vi "Pfeiffer-RVC300.get mode.vi"(0 "i ref in":refnum<vi>, 3 "ms timeout (10000)":i32=10000, 5 "error in (no error)":errorcluster) -> (14 "i ref out":refnum<vi>, 15 "regulationMode":T1, 17 "timed out":bool, 19 "error out":errorcluster)   [LabVIEW 2014, in "Pfeiffer-RVC300.lvlib"]
doc: "Gets the regulation mode from device (possible values: unknown / pressure / flow / wait).\n\nLicense Agreement for this software:\n\nCopyright (C)\nMax-Planck-Institut für Kernphysik\nSaupfercheckweg 1\n69117 Heidelberg\nGermany\n\nContact: christopher.borgmann@mpi-hd.mpg.de\n\nThis program is free software: you can redistribute it and/or modify \nit under the terms of the GNU General Public License as published by\nthe Free Software Foundation, either version 3 of the License, or\n(at your option) any later version.\n\nThis program is distributed in the hope that it will be useful,\nbut WITHOUT ANY WARRANTY; without even the implied warranty of\nMERCHANTABILITY or FITNESS FOR A PARTICULAR PURPOSE. See the\nGNU General Public License for more details.\n\nYou should have received a copy of the GNU General Public License\nalong with this program. If not, see <http://www.gnu.org/licenses/>.\n\nMax-Planck-Institut für Kernphysik\nSaupfercheckweg 1, 69117 Heidelberg, Germany\nFor all questions and ideas contact: christopher.borgmann@mpi-hd.mpg.de\nLast update: 08.07.2010"
uses:
  Pfeiffer-RVC300.lvlib
  CSCore/CSApplicationBaseClasses/DeviceBase/DeviceBase.lvlib
  Pfeiffer-RVC300.regulation mode.ctl
  CSlibraries-extern/DimLVEvent/LVDimInterface/LVDimInterface.lvlib
  CSlibraries/UtilityLib/UtilityLib.lvlib
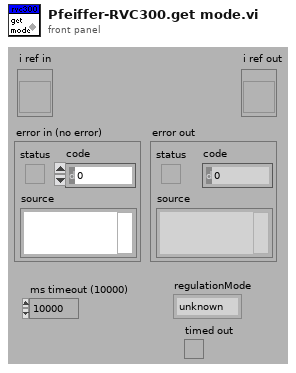
[diagram p1: front panel]
types:
  T1 = typedef "Pfeiffer-RVC300.lvlib/Pfeiffer-RVC300.regulation mode.ctl" = enum16{"unknown", "Pressure", "Flow", "Wait"}
  T2 = typedef "Pfeiffer-RVC300.lvlib/Pfeiffer-RVC300.i attribute.ctl" = cluster{"interfaceInitialized":bool, "VISAResource":refnum<visa-resource-name>, "WaitingTime":u32, "nomValues":T3, "actValues":T3}
  T3 = typedef "Pfeiffer-RVC300.lvlib/Pfeiffer-RVC300.parameters.ctl" = cluster{"regulationMode":T1, "valveType":string, "sensorType":string, "valveState":string, "flow":dbl, "pressure":dbl, "serviceIDs":cluster{"regulationModeID":i32, "valveTypeID":i32, "sensorTypeID":i32, "valveStateID":i32, "flowID":i32, "pressureID":i32}}
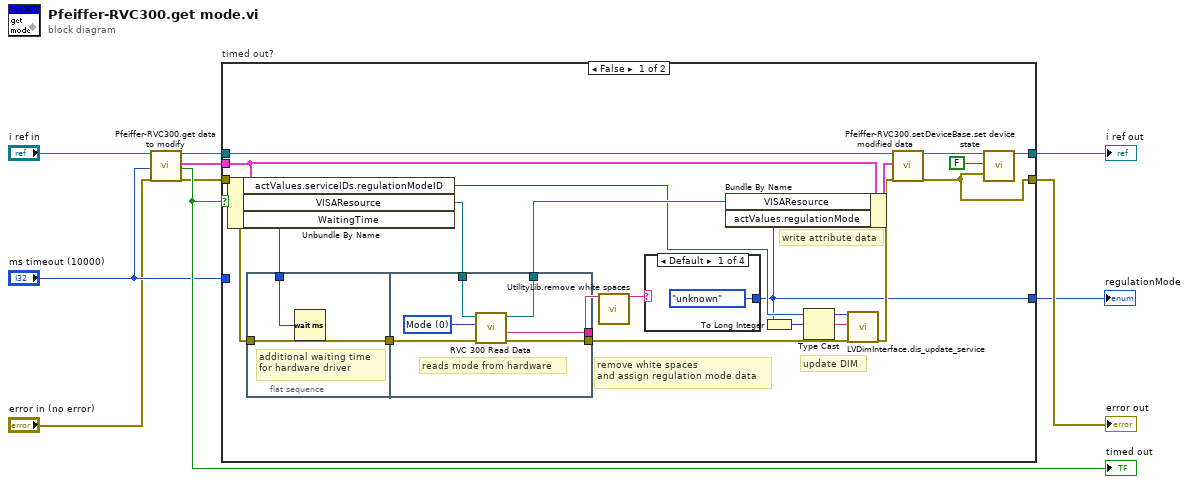
[diagram p0: block diagram]
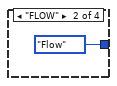
[diagram p2: hidden frame]
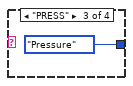
[diagram p3: hidden frame]
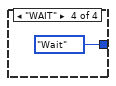
[diagram p4: hidden frame]
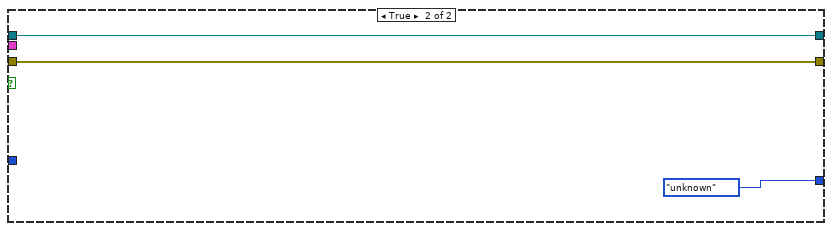
[diagram p5: hidden frame]
diagram:
  n1 = call "Pfeiffer-RVC300.get data to modify.vi"("i ref in"="i ref in", "ms timeout (10000)"="ms timeout (10000)", "error in (no error)"="error in (no error)") -> ("i ref out"=w4:refnum<vi>, "i attribute"=w2:T2, "timed out"=w7:bool, "error out"=w3:errorcluster)  [unwired: 13 in]
  "timed out" <- w7
  n2 = case "timed out?" shown="False" w7 {
    tunnel: [w27 w45] -> w9
    tunnel: w4 -> [w30 w45]
    tunnel: [w25 w44] -> w8
    tunnel: w3 -> [w24 w44]
    tunnel: w2 -> [w22 _]
    tunnel: "ms timeout (10000)" -> [_ _]
    tunnel: [w14 Pfeiffer-RVC300.regulation_mode."unknown" ("regulationMode 2")] -> w1
    frame False {
      # "write attribute data"
      # "remove white spaces\nand assign regulation mode data"
      # "update DIM"
      n3 = Unbundle By Name(w22) -> ("actValues.serviceIDs.regulationModeID"=w17:i32, "VISAResource"=w19:refnum<visa-resource-name>, "WaitingTime"=w20:u32)
      n4 = flat-sequence {
        tunnel: w24 -> [w36]
        tunnel: [w36] -> w23
        tunnel: w20 -> [w35]
        tunnel: w23 -> [w40]
        tunnel: w19 -> [w42]
        tunnel: [w39] -> w16
        tunnel: [w41] -> w21
        tunnel: [w37] -> w12
        frame #0 {
          # "additional waiting time \nfor hardware driver"
          n5 = Wait (ms)(milliseconds to wait=w35) -> ()  [unwired: 1 out]
        }
        frame #1 {
          w38 = u16 0 items=["Mode", "Pressure", "Unit", "Firmwareversion", "Keyboard lock", "Pressure Setpoint", "Sensor Type", "Valve Type"] ("RVC 300 Read")
          # "reads mode from hardware"
          n6 = call "RVC 300 Read Data.vi"("error in"=w40, "RVC 300 Read"=w38, "Resource Name"=w42) -> ("error out"=w39:errorcluster, "Response Data out"=w37:string, "Resource Name out"=w41:refnum<visa-resource-name>)  [unwired: 5 in, 1 out]
        }
      }
      n7 = call "UtilityLib.remove white spaces.vi"("string with blanks"=w12) -> ("string without white spaces"=w11:string)  [unwired: 14 in, 4 out]
      n8 = case shown="Default" w11 {
        tunnel: [Pfeiffer-RVC300.regulation_mode."unknown" Pfeiffer-RVC300.regulation_mode."Flow" Pfeiffer-RVC300.regulation_mode."Pressure" Pfeiffer-RVC300.regulation_mode."Wait"] -> w14
        frame Default {
        }
        frame "FLOW" {
        }
        frame "PRESS" {
        }
        frame "WAIT" {
        }
      }
      n9 = Bundle By Name(cluster=w22, "VISAResource"=w21, "actValues.regulationMode"=w14) -> (w29:T2)
      n10 = To Long Integer(number=w14) -> (32bit integer=w13:i32)
      n11 = Type Cast(x=w13) -> (*(type *) &x=w18:string)  [unwired: 1 in]
      n12 = call "LVDimInterface.dis_update_service.vi"("my_serviceID"=w17, "data"=w18, "error in (no error)"=w16) -> ("error out"=w15:errorcluster)  [unwired: 14 in, 2 out]
      n13 = call "Pfeiffer-RVC300.set modified data.vi"("i ref in"=w30, "i attribute"=w29, "error in (no error)"=w15) -> ("i ref out"=w28:refnum<vi>, "error out"=w25:errorcluster)  [unwired: 15 in]
      n14 = call "DeviceBase.set device state.vi"("i ref in"=w28, "implicit"=FALSE, "device error"=w25) -> ("i ref out"=w27:refnum<vi>)  [unwired: 14 in, 2 out]
    }
    frame True {
    }
  }
  "error out" <- w8
  "i ref out" <- w9
  "regulationMode" <- w1
